vi "KH7008 COM.vi"(2 "error in (no error)":errorcluster, 3 "Command":string, 4 "VISA Refnum in":refnum<visa-resource-name>="COM3") -> (0 "error out":errorcluster, 1 "Response":string="\r\n")   [LabVIEW 2013]
uses:
  <vilib>/Instr/_visa.llb/VISA Configure Serial Port (Instr).vi
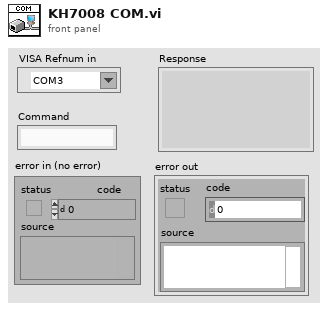
[diagram p1: front panel]
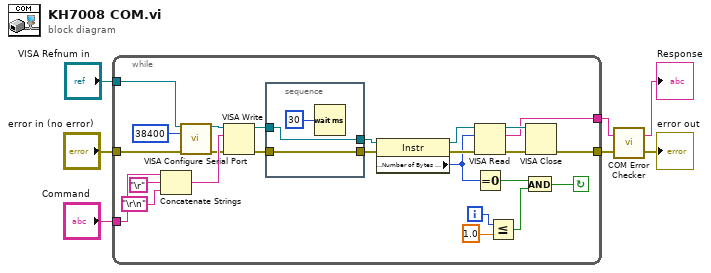
[diagram p0: block diagram]
diagram:
  n1 = while {
    tunnel: "VISA Refnum in" -> [w18]
    tunnel: "Command" -> [w17]
    tunnel: "error in (no error)" -> [w10]
    tunnel: [w9] -> w3
    tunnel: [w8] -> w4
    i -> [w14]
    stop <- w11 continue-if-true
    n2 = Concatenate Strings(w17, "\r", "\r\n") -> (w32:string)
    n3 = call-poly "VISA Configure Serial Port"("VISA resource name"=w18, "baud rate (9600)"=u32 38400 ("baud rate"), "error in (no error)"=w10) -> ("VISA resource name out"=w28:refnum<visa-resource-name>, "error out"=w29:errorcluster)  [unwired: 6 in, 5 out]
    n4 = VISA Write(VISA resource name=w28, write buffer=w32, error in (no error)=w29) -> (VISA resource name out=w24:refnum<visa-resource-name>, error out=w22:errorcluster)  [unwired: 1 out]
    n5 = stacked-sequence {
      tunnel: w22 -> [w35]
      tunnel: [w35] -> w23
      tunnel: w24 -> [w34]
      tunnel: [w34] -> w25
      frame #0 {
        n6 = Wait (ms)(milliseconds to wait=u32 30) -> ()  [unwired: 1 out]
      }
    }
    n7 = property class="Instr"(reference=w25, error in=w23) -> (reference out=w26:refnum<visa-resource-name>, error out=w27:errorcluster, "Serial Settings:Number of Bytes at Serial Port"=w16:u32)
    n8 = VISA Read(VISA resource name=w26, byte count=w16, error in (no error)=w27) -> (VISA resource name out=w21:refnum<visa-resource-name>, read buffer=w8:string, error out=w20:errorcluster)  [unwired: 1 out]
    n9 = Equal To 0?(x=w16) -> (x = 0?=w13:bool)
    n10 = Less Or Equal?(x=w14, y=1.0) -> (x <= y?=w12:bool)
    n11 = And(x=w13, y=w12) -> (x .and. y?=w11:bool)
    n12 = VISA Close(VISA resource name=w21, error in (no error)=w20) -> (error out=w9:errorcluster)
  }
  n13 = call <vilib>:"COM Error Checker.vi"("error in (no error)"=w3, "String In"=w4) -> ("error out"=→"error out":errorcluster, "String"=→"Response":string)
